vi "Element Init.vi"(7 "VolatusAPI":refnum<class "VolatusAPI.lvclass">, 8 "error in (no error)":errorcluster, 10 "JSON":string, 11 "Sequencing Control in":refnum<class "Sequencing Control.lvclass">) -> (0 "error out":errorcluster, 3 "Sequencing Control out":refnum<class "Sequencing Control.lvclass">)   [LabVIEW 2020, in "VolatusSeqGUI.lvlib" / "Sequencing Control.lvclass"]
uses:
  Sequencing Control.lvclass
  Volatus/VolatusAPI/VolatusAPI.lvclass
  Sequencing Control.lvclass/Sequencing Control.ctl
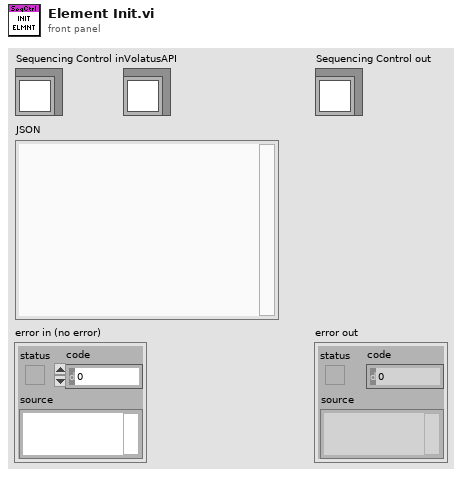
[diagram p1: front panel]
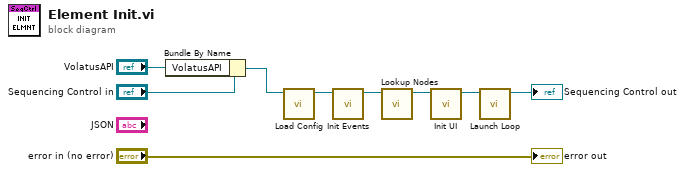
[diagram p0: block diagram]
diagram:
  n1 = Bundle By Name(cluster="Sequencing Control in", "VolatusAPI"="VolatusAPI") -> (w5:refnum<class "Sequencing Control.lvclass">)
  n2 = call "Load Config.vi"("Sequencing Control in"=w5) -> ("Sequencing Control out"=w1:refnum<class "Sequencing Control.lvclass">)  [unwired: 9 in, 1 out]
  n3 = call "Init Events.vi"("Sequencing Control in"=w1) -> ("Sequencing Control out"=w2:refnum<class "Sequencing Control.lvclass">)  [unwired: 9 in, 1 out]
  n4 = call "Lookup Nodes.vi"("Sequencing Control in"=w2) -> ("Sequencing Control out"=w7:refnum<class "Sequencing Control.lvclass">)  [unwired: 9 in, 1 out]
  n5 = call "Init UI.vi"("Sequencing Control in"=w7) -> ("Sequencing Control out"=w6:refnum<class "Sequencing Control.lvclass">)  [unwired: 9 in, 1 out]
  n6 = call "Launch Loop.vi"("Sequencing Control in"=w6) -> ("Sequencing Control out"=→"Sequencing Control out":refnum<class "Sequencing Control.lvclass">)  [unwired: 9 in, 1 out]
  "error out" <- "error in (no error)"
